vi "Update Motors.vi"(5 "Intake":dbl=-10000.0, 7 "Shooter":dbl=-10000.0, 9 "Elevator":dbl=-10000.0, 10 "Pivot":dbl=-10000.0, 11 "Climber":dbl=-10000.0) -> ()   [LabVIEW 2018]
uses:
  <vilib>/Rock Robotics/WPI/ThirdParty/Phoenix-LabVIEW/Motor Controller/Controls/CTRE_Phoenix_MotorControl_ControlMode.ctl
  Refnums.vi
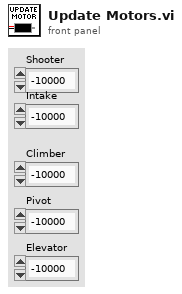
[diagram p1: front panel]
types:
  T1 = typedef "WPI_RobotDriveDevRef.ctl" = cluster{"DevStatus":errorcluster, "Motors[]":T2[], "Square Inputs":bool, "Max Output":dbl}
  T2 = typedef "WPI_MotorControlDeviceRef.ctl" = cluster{"DeviceStatus":errorcluster, "Type":T3, "PWM":cluster{"PWM Channel":T4, "DeadBand":T5}, "CAN":cluster{"Device Number":u8, "SetOutput VI Ref":variant, "GetOutput VI Ref":variant, "Enable VI Ref":variant, "Disable VI Ref":variant, "Data":variant}, "Invert":bool, "DIO PWM":cluster{"PWM \"Enable\" Channel":T4, "DIOChannel":T6, "PWM Rate":dbl}}
  T3 = typedef "WPI_MotorControlType.ctl" = enum16{"PWM", "CAN", "DIO PWM"}
  T4 = typedef "FPGA_DIOPWMChannel.ctl" = enum8{"PWM 0", "PWM 1", "PWM 2", "PWM 3", "PWM 4", "PWM 5", "PWM 6", "PWM 7", "PWM 8", "PWM 9", "PWM MXP 0", "PWM MXP 1", "PWM MXP 2", "PWM MXP 3", "PWM MXP 4", "PWM MXP 5", "PWM MXP 6", "PWM MXP 7", "PWM MXP 8", "PWM MXP 9", "Invalid"}
  T5 = typedef "WPI_PWMDeadband.ctl" = cluster{"Name":string, "maxPositivePwm":i32, "minPositivePwm":i32, "centerPwm":i32, "maxNegativePwm":i32, "minNegativePwm":i32, "angularRange":u16}
  T6 = typedef "FPGA_DIOChannel.ctl" = enum8{"DIO 0", "DIO 1", "DIO 2", "DIO 3", "DIO 4", "DIO 5", "DIO 6", "DIO 7", "DIO 8", "DIO 9", "DIO MXP 0", "DIO MXP 1", "DIO MXP 2", "DIO MXP 3", "DIO MXP 4", "DIO MXP 5", "DIO MXP 6", "DIO MXP 7", "DIO MXP 8", "DIO MXP 9", "DIO MXP 10", "DIO MXP 11", "DIO MXP 12", "DIO MXP 13", "DIO MXP 14", "DIO MXP 15", "SPI Port CS1", "SPI Port CS2", "SPI Port CS3", "SPI Port MISO", "SPI Port MOSI", "Invalid"}
  T7 = cluster{"DriveTrain":T1, "LeftDrive":T2, "RightDrive":T2, "Elevator":T2, "Pivot":T2, "Intake":T2, "Right Climber":T2, "Left Climber":T2, "Shooter":T2}
  T8 = typedef "CTRE_Phoenix_MotorControl_ControlMode.ctl" = u16
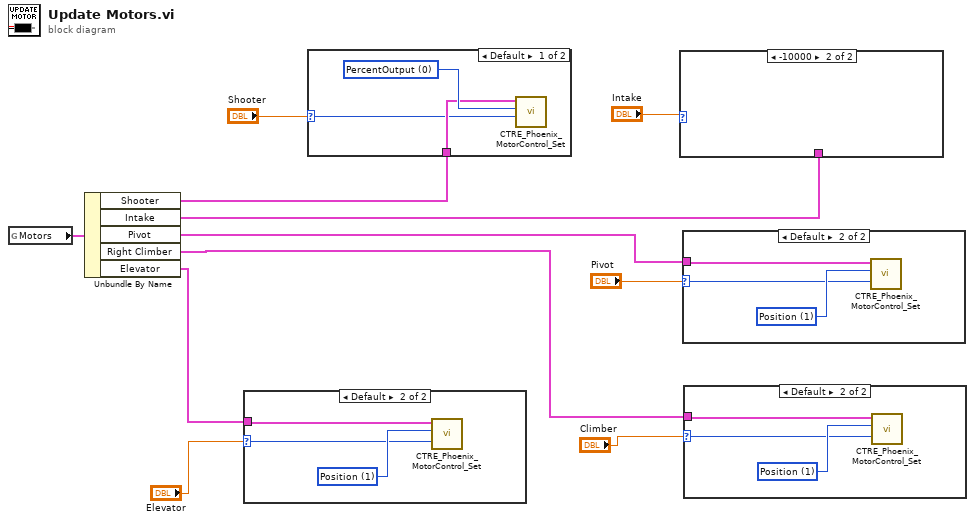
[diagram p0: block diagram]
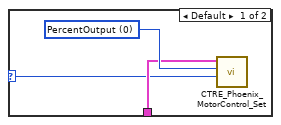
[diagram p5: hidden frame]
diagram:
  n1 = global read "Refnums.vi" "Motors"() -> (w11:T7)
  n2 = Unbundle By Name(w11) -> ("Shooter"=w10:T2, "Intake"=w7:T2, "Pivot"=w9:T2, "Right Climber"=w4:T2, "Elevator"=w2:T2)
  n3 = case shown="Default" "Elevator" {
    selector: "Elevator" -> [_ w12]
    tunnel: w2 -> [_ w13]
    frame -10000 {
    }
    frame Default {
      w14 = T8 1 items=["PercentOutput"=0, "Position"=1, "Velocity"=2, "Current"=3, "Follower"=5, "MotionProfile"=6, "MotionMagic"=7, "MotionProfileArc"=10, "Disabled"=15] ("Control Mode")
      n4 = call <vilib>:"CTRE_Phoenix_MotorControl_Set.vi"("Output"=w12, "Control Mode"=w14, "PhoenixMotorControlDevRef"=w13) -> ()  [unwired: 7 in, 2 out]
    }
  }
  n5 = case shown="Default" "Shooter" {
    selector: "Shooter" -> [w15 _]
    tunnel: w10 -> [w16 _]
    frame Default {
      w17 = T8 0 items=["PercentOutput"=0, "Position"=1, "Velocity"=2, "Current"=3, "Follower"=5, "MotionProfile"=6, "MotionMagic"=7, "MotionProfileArc"=10, "Disabled"=15] ("Control Mode")
      n6 = call <vilib>:"CTRE_Phoenix_MotorControl_Set.vi"("Output"=w15, "Control Mode"=w17, "PhoenixMotorControlDevRef"=w16) -> ()  [unwired: 7 in, 2 out]
    }
    frame -10000 {
    }
  }
  n7 = case shown="-10000" "Intake" {
    selector: "Intake" -> [w18 _]
    tunnel: w7 -> [w19 _]
    frame Default {
      w20 = T8 0 items=["PercentOutput"=0, "Position"=1, "Velocity"=2, "Current"=3, "Follower"=5, "MotionProfile"=6, "MotionMagic"=7, "MotionProfileArc"=10, "Disabled"=15] ("Control Mode")
      n8 = call <vilib>:"CTRE_Phoenix_MotorControl_Set.vi"("Output"=w18, "Control Mode"=w20, "PhoenixMotorControlDevRef"=w19) -> ()  [unwired: 7 in, 2 out]
    }
    frame -10000 {
    }
  }
  n9 = case shown="Default" "Pivot" {
    selector: "Pivot" -> [_ w21]
    tunnel: w9 -> [_ w22]
    frame -10000 {
    }
    frame Default {
      w23 = T8 1 items=["PercentOutput"=0, "Position"=1, "Velocity"=2, "Current"=3, "Follower"=5, "MotionProfile"=6, "MotionMagic"=7, "MotionProfileArc"=10, "Disabled"=15] ("Control Mode")
      n10 = call <vilib>:"CTRE_Phoenix_MotorControl_Set.vi"("Output"=w21, "Control Mode"=w23, "PhoenixMotorControlDevRef"=w22) -> ()  [unwired: 7 in, 2 out]
    }
  }
  n11 = case shown="Default" "Climber" {
    selector: "Climber" -> [_ w24]
    tunnel: w4 -> [_ w25]
    frame -10000 {
    }
    frame Default {
      w26 = T8 1 items=["PercentOutput"=0, "Position"=1, "Velocity"=2, "Current"=3, "Follower"=5, "MotionProfile"=6, "MotionMagic"=7, "MotionProfileArc"=10, "Disabled"=15] ("Control Mode")
      n12 = call <vilib>:"CTRE_Phoenix_MotorControl_Set.vi"("Output"=w24, "Control Mode"=w26, "PhoenixMotorControlDevRef"=w25) -> ()  [unwired: 7 in, 2 out]
    }
  }
